vi "Coral Target Loop.vi"(0 "Camera Name":string="cam0") -> ()   [LabVIEW 2023]
uses:
  April Tags/Camera Info.ctl
  State Machine/Coral States.ctl
  State Machine/Coral Main CLuster.ctl
  <vilib>/vision/Image Controls.llb/IMAQ Image.ctl
  Steam Type.ctl
  Ball/State Machine/Ball States.ctl
  Camera Set Up/Event Setup Types.ctl
  <vilib>/Rock Robotics/Network Tables/NT Write String.vi
  <vilib>/Utility/config.llb/Read Key (String).vi
  <vilib>/Utility/config.llb/Write Key (String).vi
  <vilib>/Utility/config.llb/NI_LVConfig.lvlib
  <vilib>/vision/NI_Vision_Development_Module.lvlib
panel:
  in  "Main":enum32{"Page 1", "Page 2"}(tab)
  out "Algae Distance":dbl[](array[numeric]) caption="Distance" format="%.1f"
  out "Algae Angle":dbl[](array[numeric]) caption="Angle" format="%.1f"
  out "Image":T1(plugin-control)
  in  "Settings":bool
  in  "Save":bool
  in  "Tools":bool
  out "Ball Fps":dbl format="%#.0f"
  in  "Home":bool
  in  "FOV":dbl=68.5
  in  "Coral Color Range":T2={"Hue"={21.620689392089844, 69.62068939208984}, "Sat"={66.41378784179688, 255.0}, "Val"={96.0, 255.0}} caption="Color Range" {"Hue" scale=0.0..255.0 scale format="%#_3g"}
  out "Mask":T1(plugin-control)
  in  "Score Threshold %":dbl=80.0
  in  "Robot Calibration Cluster":T3={"Camera Height on robot (in)"=34.5, "Camera Angle on the robot (deg)"=28.3, "Camera FOV Top to Bottom View Angle (deg)"=0.946, "Camera FOV Left to Right View Angle (deg)"=26.5, "Target size (in)"=6.5, "Distance to front of bumper (in)"=9.75, "Focal Length (mm)"=10.0} {"Camera FOV Left to Right View Angle (deg)" format="%#_13g"; "Focal Length (mm)" format="%#_13g"; "Distance to front of bumper (in)" format="%#_13g"; "Target size (in)" format="%#_13g"; "Camera FOV Top to Bottom View Angle (deg)" format="%#_13g"; "Camera Angle on the robot (deg)" format="%#_13g"; "Camera Height on robot (in)" format="%#_13g"}
  # "Edit the camera name to the camera that you are going to use for this target package"
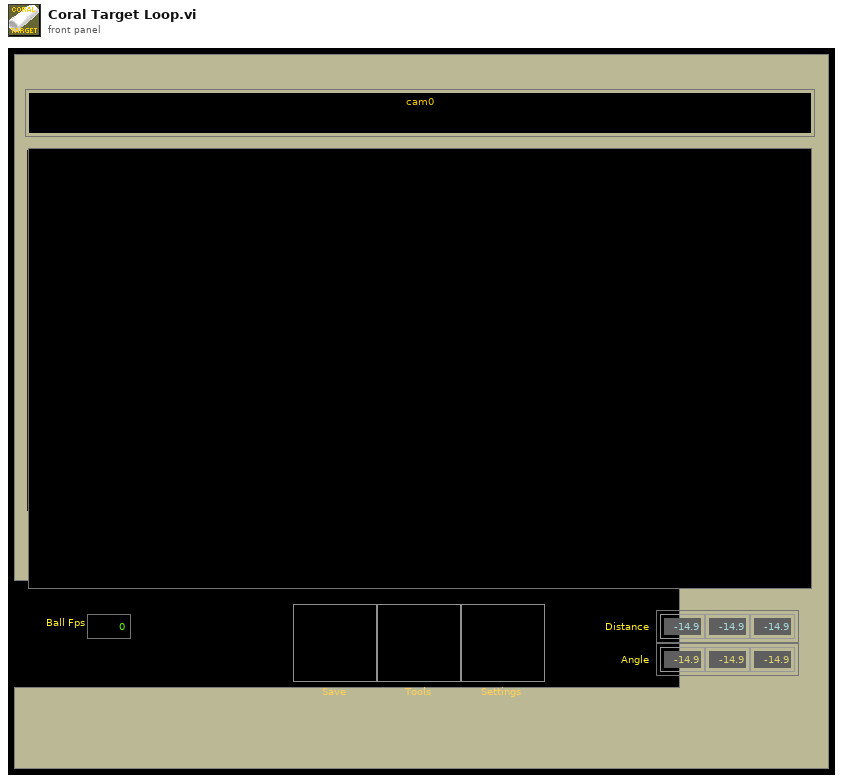
[diagram p1: front panel]
types:
  T1 = typedef "IMAQ Image.ctl" = refnum<image>
  T2 = cluster{"Hue":cluster{dbl, dbl}, "Sat":cluster{dbl, dbl}, "Val":cluster{dbl, dbl}}
  T3 = typedef "Camera Info.ctl" = cluster{"Camera Height on robot (in)":dbl, "Camera Angle on the robot (deg)":dbl, "Camera FOV Top to Bottom View Angle (deg)":dbl, "Camera FOV Left to Right View Angle (deg)":dbl, "Target size (in)":dbl, "Distance to front of bumper (in)":dbl, "Focal Length (mm)":dbl}
  T4 = typedef "Coral Main CLuster.ctl" = cluster{"Coral FIFO":T5[], "Camera Name":string, "Coral path":path, "Control Ref's":refnum<vi>[], "Greyscale Mask Image":T1, "Main Image":T1, "Coral Color Range":cluster{"Hue":cluster{dbl, dbl}, "Sat":cluster{dbl, dbl}, "Val":cluster{dbl, dbl}}, "Timeout":i32}
  T5 = typedef "Coral States.ctl" = enum16{"Message Dispatcher", "INI", "Open", "Save", "Exit"}
  T6 = typedef "Particle Parameters" = i32
  T7 = typedef "Steam Type.ctl" = enum8{"Unknown", "Apriltag", "Algae", "Coral"}
  T8 = typedef "Event Setup Types.ctl" = enum16{"Default", "Camera Loop Started", "Close Settings", "GreyScale", "Open Front Panel", "Save Data", "Exit"}
  T9 = typedef "Ball States.ctl" = enum16{"Message Dispatcher", "INI", "Open", "Save", "Exit"}
  T10 = typedef "Target Fields.ctl" = cluster{"diameter points":cluster{"first point":cluster{"x":dbl, "y":dbl}, "projected point":cluster{"x":dbl, "y":dbl}}, "normalized center":cluster{"x":dbl, "y":dbl}, "Overall Score":dbl, "Area Score":dbl, "Moment Score":dbl, "Aspect Score":dbl, "Distance (ft)":dbl, "Upper Goal":bool}
  T11 = cluster{cluster{"Lower":dbl, "Upper":dbl}, cluster{"Lower":dbl, "Upper":dbl}, cluster{"Lower":dbl, "Upper":dbl}}
  T12 = typedef "Image Type" = u32
  T13 = typedef "NI_LVConfig.lvlib/Config Data RefNum.ctl" = refnum<k1>
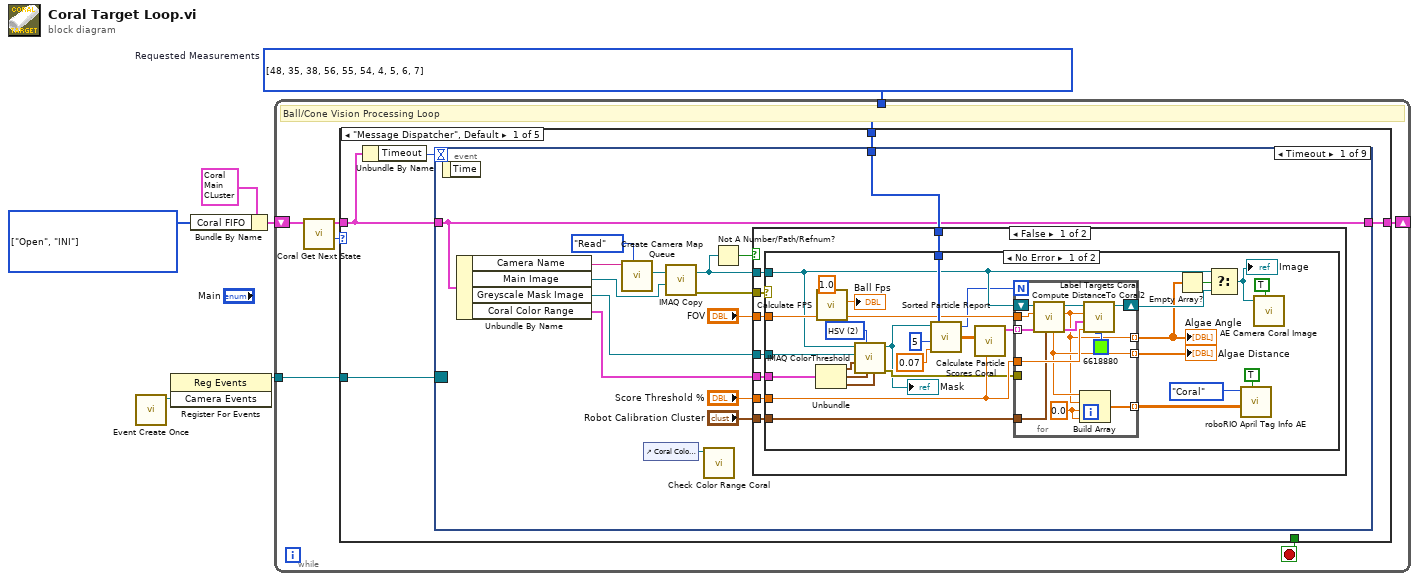
[diagram p0: block diagram]
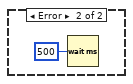
[diagram p2: hidden frame]
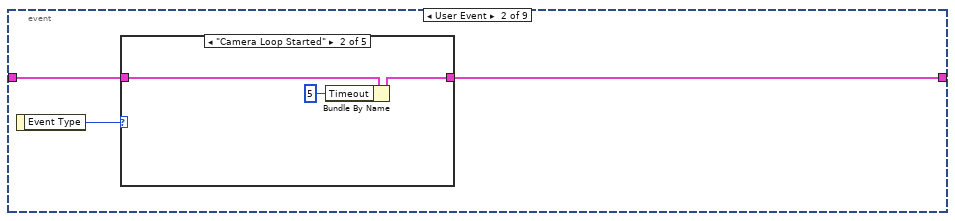
[diagram p4: hidden frame]
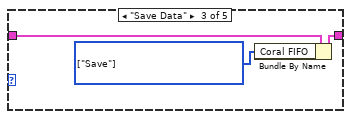
[diagram p6: hidden frame]
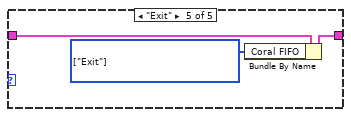
[diagram p8: hidden frame]
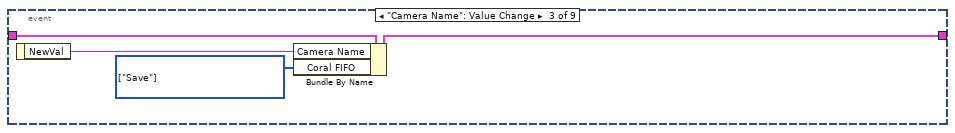
[diagram p9: hidden frame]
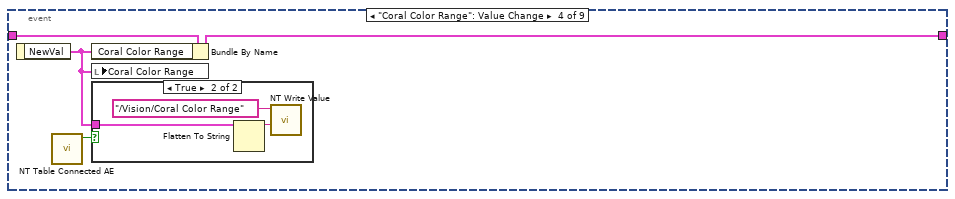
[diagram p10: hidden frame]
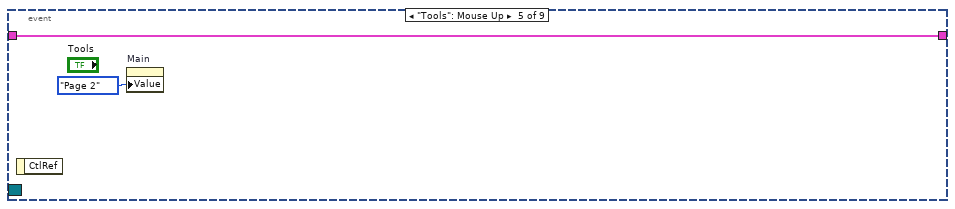
[diagram p12: hidden frame]
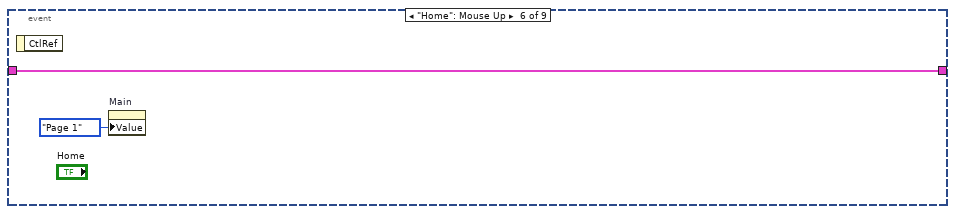
[diagram p13: hidden frame]
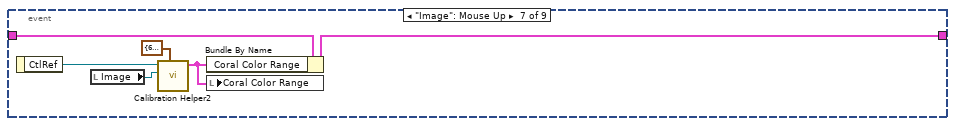
[diagram p14: hidden frame]
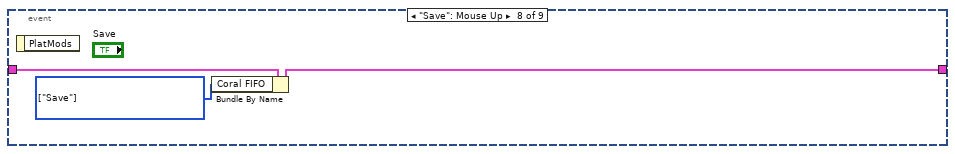
[diagram p15: hidden frame]
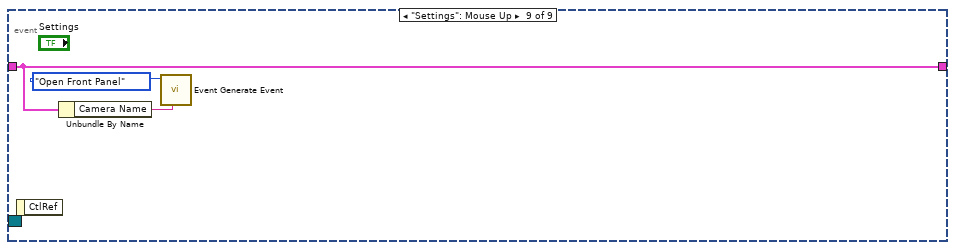
[diagram p16: hidden frame]
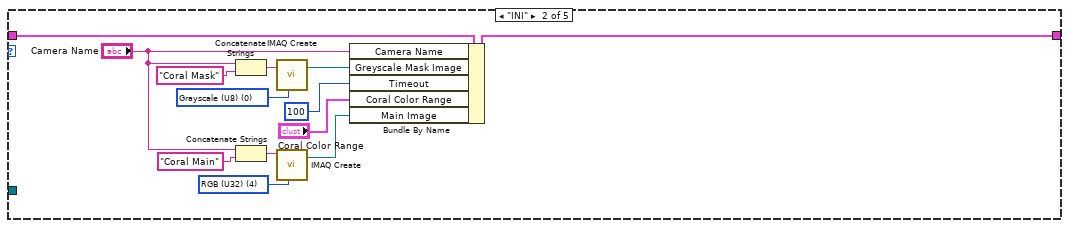
[diagram p17: hidden frame]
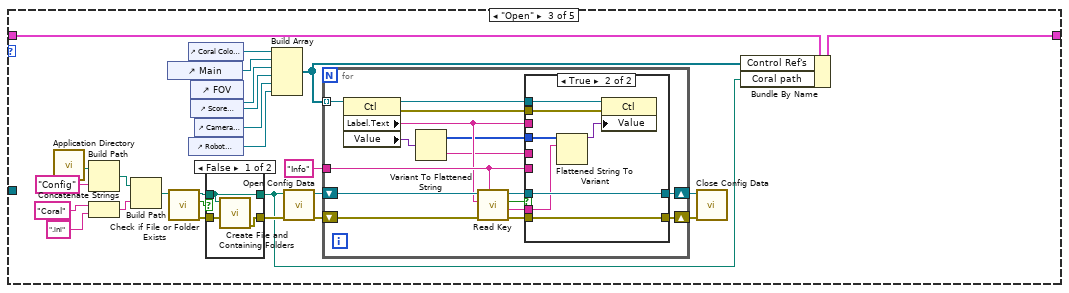
[diagram p18: hidden frame]
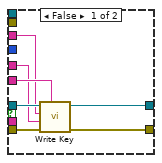
[diagram p20: hidden frame]
diagram:
  w2 = T5[] [enum."Open", enum."INI"] items=["Message Dispatcher", "INI", "Open", "Save", "Exit"] ("Ball FIFO")
  w4 = T6[] [48, 35, 38, 56, 55, 54, 4, 5, 6, 7] items=["Center of Mass X", "Center of Mass Y", "First Pixel X", "First Pixel Y", "Bounding Rect Left", "Bounding Rect Top", "Bounding Rect Right", "Bounding Rect Bottom", "Max Feret Diameter Start X", "Max Feret Diameter Start Y", "Max Feret Diameter End X", "Max Feret Diameter End Y", "Max Horiz. Segment Length Left", "Max Horiz. Segment Length Right", "Max Horiz. Segment Length Row", "-", "Bounding Rect Width", "Bounding Rect Height", "Bounding Rect Diagonal", "Perimeter", "Convex Hull Perimeter", "Holes' Perimeter", "Max Feret Diameter", "Equivalent Ellipse Major Axis", "Equivalent Ellipse Minor Axis", "Equivalent Ellipse Minor Axis (Feret)", "Equivalent Rect Long Side", "Equivalent Rect Short Side", "Equivalent Rect Diagonal", "Equivalent Rect Short Side (Feret)", "Average Horiz. Segment Length", "Average Vert. Segment Length", "Hydraulic Radius", "Waddel Disk Diameter", "-", "Area", "Holes' Area", "Particle & Holes' Area", "Convex Hull Area", "Image Area", "-", "Number of Holes", "Number of Horiz. Segments", "Number of Vert. Segments", "-", "Orientation", "Max Feret Diameter Orientation", "-", "% Area/Image Area", "% Area/(Particle & Holes' Area)", "Ratio of Equivalent Ellipse Axes", "Ratio of Equivalent Rect Sides", "-", "Elongation Factor", "Compactness Factor", "Heywood Circularity Factor", "Type Factor", "-", "Sum X", "Sum Y", "Sum XX", "Sum XY", "Sum YY", "Sum XXX", "Sum XXY", "Sum XYY", "Sum YYY", "-", "Moment of Inertia XX", "Moment of Inertia XY", "Moment of Inertia YY", "Moment of Inertia XXX", "Moment of Inertia XXY", "Moment of Inertia XYY", "Moment of Inertia YYY", "Norm. Moment of Inertia XX", "Norm. Moment of Inertia XY", "Norm. Moment of Inertia YY", "Norm. Moment of Inertia XXX", "Norm. Moment of Inertia XXY", "Norm. Moment of Inertia XYY", "Norm. Moment of Inertia YYY", "Hu Moment 1", "Hu Moment 2", "Hu Moment 3", "Hu Moment 4", "Hu Moment 5", "Hu Moment 6", "Hu Moment 7"]  # Requested Measurements
  n1 = call "Event Create Once.vi"() -> ("Camera Events"=w6:refnum<user-event>)  [unwired: 10 in, 1 out]
  n2 = register-events(w6) -> (reference out=w5:refnum<event-registration>)  [unwired: 2 in, 1 out]
  n3 = Bundle By Name(cluster=T4 {"Coral FIFO"=[], "Camera Name"="", "Coral path"=path "", "Control Ref's"=[], "Greyscale Mask Image"=refnum, "Main Image"=refnum, "Coral Color Range"={"Hue"={21.620689392089844, 69.62068939208984}, "Sat"={66.41378784179688, 255.0}, "Val"={96.0, 255.0}}, "Timeout"=5} ("output cluster"), "Coral FIFO"=w2) -> (w3:T4)
  n4 = while {
    tunnel: w4 -> [w13]
    tunnel: w5 -> [w12]
    shift-right: [w7] -> _
    shift-left: w3 -> [w10]
    stop <- w11 stop-if-true
    # "Ball/Cone Vision Processing Loop"
    n5 = call "Coral Get Next State.vi"("Coral Main Cluster in"=w10) -> ("Next State"=w9:T9, "Coral Main Cluster out"=w8:T4)  [unwired: 9 in]
    n6 = case shown="\"Message Dispatcher\", Default" w9 {
      tunnel: w13 -> [w18 _ _ _ _]
      tunnel: w12 -> [w17 _ _ _ _]
      tunnel: [_ _ _ _ TRUE] -> w11
      tunnel: w8 -> [w15 w135 w149 w202 w219]
      tunnel: [w16 w134 w147 w202 w219] -> w7
      frame "Message Dispatcher", Default {
        n7 = Unbundle By Name(w15) -> ("Timeout"=w14:i32)
        n8 = event shown="[0] Timeout" {
          selector: w17 -> [_ _ _ _ _ _ _ _ _]
          dyn-events: _ -> [_ _ _ _ _ _ _ _ _]
          timeout: w14 -> [_ _ _ _ _ _ _ _ _]
          tunnel: w18 -> [w33 _ _ _ _ _ _ _ _]
          tunnel: w15 -> [w28 w87 w102 w106 w110 w112 w116 w122 w124]
          tunnel: [w28 w85 w101 w105 w110 w112 w115 w121 w124] -> w16
          event Timeout {
            n9 = event-data() -> ()  [unwired: 1 in, 1 out]
            n10 = Unbundle By Name(w28) -> ("Camera Name"=w30:string, "Main Image"=w24:T1, "Greyscale Mask Image"=w29:T1, "Coral Color Range"=w27:T2)
            n11 = call "Create Camera Map Queue.vi"("Action"=enum16{"Read", "Write"}."Read", "Camera"=w30) -> ("Image out"=w25:T1)  [unwired: 8 in, 1 out]
            n12 = control-ref of="Coral Color Range"() -> (w21:refnum<vi>)
            n13 = call "IMAQ Copy"("Image Dst"=w24, "Image Src"=w25) -> ("error out"=w23:errorcluster, "Image Dst Out"=w19:T1)  [unwired: 4 in]
            n14 = call "Check Color Range Coral.vi"("Coral Color Range"=w21) -> ()  [unwired: 11 in]
            n15 = Not A Number/Path/Refnum?(number/path/refnum=w19) -> (NaN/Path/Refnum?=w20:bool)
            n16 = case shown="False" w20 {
              tunnel: w33 -> [w41 _]
              tunnel: "Score Threshold %" -> [w40 _]
              tunnel: w29 -> [w39 _]
              tunnel: w27 -> [w38 _]
              tunnel: "FOV" -> [w37 _]
              tunnel: w19 -> [w36 _]
              tunnel: w23 -> [w35 _]
              tunnel: "Robot Calibration Cluster" -> [w34 _]
              frame False {
                n17 = case shown="No Error" w35 {
                  tunnel: w41 -> [w70 _]
                  tunnel: w39 -> [w68 _]
                  tunnel: w37 -> [w67 _]
                  tunnel: w38 -> [w66 _]
                  tunnel: w40 -> [w65 _]
                  tunnel: w36 -> [w64 _]
                  tunnel: w34 -> [w43 _]
                  frame No Error {
                    w59 = u16 2 items=["RGB", "HSL", "HSV", "HSI"] ("Color Mode")
                    n18 = Unbundle(w66) -> ("Hue"=w54:cluster{dbl, dbl}, "Sat"=w53:cluster{dbl, dbl}, "Val"=w52:cluster{dbl, dbl})
                    n19 = call "Calculate FPS.vi"("Frames Processed"=1.0) -> ("Fps"=→"Ball Fps":dbl)  [unwired: 10 in]
                    n20 = call "IMAQ ColorThreshold"("Blue or Luma or Val or Inten Range"=w52, "Green or Sat Range"=w53, "Color Mode"=w59, "Red or Hue Range"=w54, "Image Dst"=w68, "Image Src"=w64) -> ("error out"=w58:errorcluster, "Image Dst Out"=w42:T1)  [unwired: 4 in]
                    "Mask" <- w42
                    n21 = call "Sorted Particle Report.vi"("Min Area Size %"=0.07 ("Size Limit %"), "Particle Count Limit"=5 ("Particle Count LImit"), "Pixel Measurements"=w70, "Image in"=w42) -> ("Sorted Data"=w62:dbl[][], "Particles"=w57:i32)  [unwired: 1 out]
                    n22 = call "Calculate Particle Scores Coral.vi"("Limit"=w65, "Sorted Data"=w62) -> ("Scores"=w61:T10[])  [unwired: 9 in]
                    n23 = for {
                      N: w57 -> [_]
                      tunnel: w61 -> [w81] mode=indexing
                      shift-right: [w83] -> w56
                      shift-left: w64 -> [w79]
                      tunnel: w65 -> [w82]
                      tunnel: [w74] -> w51 mode=indexing
                      tunnel: w58 -> [_]
                      tunnel: w67 -> [w77]
                      tunnel: [w75] -> w50 mode=indexing
                      tunnel: [w72] -> w44 mode=indexing
                      tunnel: w43 -> [w71]
                      w73 = 0.0 ("element")
                      n24 = call "Compute DistanceTo Coral2.vi"("Robot Calibration Cluster"=w71, "results 2"=w81, "FOV Left to Right (deg)"=w77, "Image Src"=w79) -> ("results out"=w78:T10, "Offset Angle"=w74:dbl, "Image Dst Out"=w80:T1, "Distance from target (in)"=w75:dbl)  [unwired: 4 in]
                      n25 = Build Array(w75, w74, w73, w73) -> (w72:dbl[])
                      n26 = call "Label Targets Coral.vi"("Color"=u32 6618880, "Score Threshold"=w82, "results"=w78, "Angle"=w74, "Image in"=w80) -> ("Image out"=w83:T1)  [unwired: 6 in]
                    }
                    "Algae Angle" <- w51
                    "Algae Distance" <- w50
                    n27 = Empty Array?(array=w51) -> (empty?=w55:bool)
                    n28 = Select(t=w64, s=w55, f=w56) -> (s? t:f=w69:T1)
                    "Image" <- w69
                    n29 = call "roboRIO April Tag Info AE.vi"("Update"=TRUE, "Info in"=w44, "Stream Type"=Steam_Type."Coral") -> ()  [unwired: 8 in, 1 out]
                    n30 = call "AE Camera Coral Image.vi"("Update"=TRUE, "Ball Image in"=w69) -> ()  [unwired: 9 in, 1 out]
                  }
                  frame Error {
                    n31 = Wait (ms)(milliseconds to wait=u32 500) -> ()  [unwired: 1 out]
                  }
                }
              }
              frame True {
              }
            }
          }
          event User Event {
            n32 = event-data() -> ("Event Type"=w86:T8)  [unwired: 1 in]
            n33 = case shown="\"Camera Loop Started\"" w86 {
              tunnel: w87 -> [w88 w91 w94 w95 w98]
              tunnel: [w88 w90 w93 w95 w97] -> w85
              frame "Default", Default {
              }
              frame "Camera Loop Started" {
                n34 = Bundle By Name(cluster=w91, "Timeout"=5) -> (w90:T4)
              }
              frame "Save Data" {
                w92 = T9[] [enum."Save"] items=["Message Dispatcher", "INI", "Open", "Save", "Exit"] ("Ball FIFO")
                n35 = Bundle By Name(cluster=w94, "Coral FIFO"=w92) -> (w93:T4)
              }
              frame "Open Front Panel" {
              }
              frame "Exit" {
                w96 = T9[] [enum."Exit"] items=["Message Dispatcher", "INI", "Open", "Save", "Exit"] ("Ball FIFO")
                n36 = Bundle By Name(cluster=w98, "Coral FIFO"=w96) -> (w97:T4)
              }
            }
          }
          event "Camera Name": Value Change {
            w99 = T9[] [enum."Save"] items=["Message Dispatcher", "INI", "Open", "Save", "Exit"] ("Ball FIFO")
            n37 = event-data() -> ("NewVal"=w100:string)  [unwired: 1 in]
            n38 = Bundle By Name(cluster=w102, "Camera Name"=w100, "Coral FIFO"=w99) -> (w101:T4)
          }
          event "Coral Color Range": Value Change {
            n39 = event-data() -> ("NewVal"=w103:T2)  [unwired: 1 in]
            n40 = call "NT Table Connected AE.vi"() -> ("NT Table Connected out"=w104:bool)  [unwired: 11 in]
            n41 = Bundle By Name(cluster=w106, "Coral Color Range"=w103) -> (w105:T4)
            n42 = local write "Coral Color Range"(w103) -> ()
            n43 = case shown="True" w104 {
              tunnel: w103 -> [_ w107]
              frame False {
              }
              frame True {
                n44 = Flatten To String(anything=w107) -> (data string=w109:string)  [unwired: 3 in, 2 out]
                n45 = call-poly <vilib>:"NT Write Value.vi"("value"=w109, "name"="/Vision/Coral Color Range" ("Name")) -> ()  [unwired: 9 in, 1 out]
              }
            }
          }
          event "Tools": Mouse Up {
            n46 = event-data() -> ()  [unwired: 1 in, 1 out]
            n47 = property on="Main" class="TabCtl (strict)"("Value"=enum32{"Page 1", "Page 2"}."Page 2" ("Main")) -> ()  [unwired: 2 in, 2 out]
          }
          event "Home": Mouse Up {
            n48 = event-data() -> ()  [unwired: 1 in, 1 out]
            n49 = property on="Main" class="TabCtl (strict)"("Value"=enum32{"Page 1", "Page 2"}."Page 1" ("Main")) -> ()  [unwired: 2 in, 2 out]
          }
          event "Image": Mouse Up {
            n50 = event-data() -> ("CtlRef"=w118:refnum<vi>)  [unwired: 1 in]
            n51 = local read "Image"() -> (w117:T1)
            n52 = call "Calibration Helper2.vi"("Std Devs"=cluster{"H":dbl, "S":dbl, "V":dbl} {"H"=6.0, "S"=6.0, "V"=6.0} ("Std Devs Ball"), "Image"=w117, "Image Ctl Refnum"=w118) -> ("output color"=w114:T11)  [unwired: 7 in, 1 out]
            n53 = Bundle By Name(cluster=w116, "Coral Color Range"=w114) -> (w115:T4)
            n54 = local write "Coral Color Range"(w114) -> ()
          }
          event "Save": Mouse Up {
            w120 = T9[] [enum."Save"] items=["Message Dispatcher", "INI", "Open", "Save", "Exit"] ("Ball FIFO")
            n55 = event-data() -> ()  [unwired: 1 in, 1 out]
            n56 = Bundle By Name(cluster=w122, "Coral FIFO"=w120) -> (w121:T4)
          }
          event "Settings": Mouse Up {
            n57 = event-data() -> ()  [unwired: 1 in, 1 out]
            n58 = Unbundle By Name(w124) -> ("Camera Name"=w123:string)
            n59 = call "Event Generate Event.vi"("Camera Name"=w123, "Event Type"=Event_Setup_Types."Open Front Panel") -> ()  [unwired: 10 in]
          }
        }
      }
      frame "INI" {
        w131 = T12 4 items=["Grayscale (U8)", "Grayscale (I16)", "Grayscale (SGL)", "Complex (CSG)", "RGB (U32)", "HSL (U32)", "RGB (U64)", "Grayscale (U16)"] ("Image Type")
        w136 = T12 0 items=["Grayscale (U8)", "Grayscale (I16)", "Grayscale (SGL)", "Complex (CSG)", "RGB (U32)", "HSL (U32)", "RGB (U64)", "Grayscale (U16)"] ("Image Type")
        n60 = Concatenate Strings("Camera Name", "Coral Mask" ("string")) -> (w138:string)
        n61 = Concatenate Strings("Camera Name", "Coral Main" ("string")) -> (w130:string)
        n62 = call "IMAQ Create"("Image Name"=w138, "Image Type"=w136) -> ("New Image"=w133:T1)  [unwired: 2 in, 2 out]
        n63 = call "IMAQ Create"("Image Name"=w130, "Image Type"=w131) -> ("New Image"=w127:T1)  [unwired: 2 in, 2 out]
        n64 = Bundle By Name(cluster=w135, "Camera Name"="Camera Name", "Greyscale Mask Image"=w133, "Timeout"=100, "Coral Color Range"="Coral Color Range", "Main Image"=w127) -> (w134:T4)
      }
      frame "Open" {
        n65 = call <vilib>:"Application Directory.vi"() -> ("Application Directory"=w152:path)
        n66 = Build Path(base path=w152, name or relative path="Config") -> (appended path=w150:path)
        n67 = Concatenate Strings("Coral" ("string"), ".ini" ("name or relative path")) -> (w164:string)
        n68 = Build Path(base path=w150, name or relative path=w164) -> (appended path=w145:path)
        n69 = control-ref of="Main"() -> (w157:refnum<vi>)
        n70 = call <vilib>:"Check if File or Folder Exists.vi"("path"=w145) -> ("error out"=w141:errorcluster, "file or folder exists?"=w143:bool, "dup path"=w144:path)  [unwired: 8 in]
        n71 = control-ref of="Coral Color Range"() -> (w158:refnum<vi>)
        n72 = control-ref of="Robot Calibration Cluster"() -> (w139:refnum<vi>)
        n73 = control-ref of="FOV"() -> (w156:refnum<vi>)
        n74 = control-ref of="Score Threshold %"() -> (w155:refnum<vi>)
        n75 = control-ref of="Camera Name"() -> (w140:refnum<vi>)
        n76 = case shown="False" w143 {
          tunnel: [w167 w168] -> w153
          tunnel: w144 -> [w166 w169]
          tunnel: [w166 w169] -> w142
          tunnel: w141 -> [w165 w168]
          frame False {
            n77 = call <vilib>:"Create File and Containing Folders.vi"("error in (no error)"=w165, "file path"=w166) -> ("error out"=w167:errorcluster)  [unwired: 8 in, 1 out]
          }
          frame True {
          }
        }
        n78 = Build Array(w158, w157, w156, w155, w140, w139) -> (w146:refnum<vi>[])
        n79 = call <vilib>:"Open Config Data.vi"("error in (no error)"=w153, "configuration file path"=w142) -> ("error out"=w159:errorcluster, "refnum"=w163:T13)  [unwired: 7 in, 1 out]
        n80 = for {
          tunnel: "Info" ("Camera Name") -> [w182]
          tunnel: w146 -> [w172] mode=indexing
          shift-right: [w184] -> w162
          shift-left: w163 -> [w185]
          shift-right: [w183] -> w161
          shift-left: w159 -> [w181]
          n81 = property class="Ctl"(reference=w172) -> (reference out=w178:refnum<vi>, error out=w177:errorcluster, "Label.Text"=w175:string, "Value"=w171:variant)  [unwired: 1 in]
          n82 = Variant To Flattened String(Variant=w171) -> (data string=w173:string, 1:w170:i16[])
          n83 = call-poly <vilib>:"Read Key.vi"("section"=w182, "error in (no error)"=w181, "key"=w175, "refnum"=w185) -> ("error out"=w174:errorcluster, "value"=w179:string, "found?"=w180:bool, "refnum out"=w176:T13)  [unwired: 4 in]
          n84 = case shown="True" w180 {
            tunnel: w179 -> [_ w194]
            tunnel: w178 -> [_ w199]
            tunnel: w177 -> [_ w198]
            tunnel: w176 -> [w192 w197]
            tunnel: w182 -> [w191 _]
            tunnel: w175 -> [w190 _]
            tunnel: [w189 w197] -> w184
            tunnel: w174 -> [w188 w196]
            tunnel: [w187 w196] -> w183
            tunnel: w173 -> [w186 _]
            tunnel: w170 -> [_ w193]
            frame False {
              n85 = call-poly <vilib>:"Write Key.vi"("section"=w191, "error in (no error)"=w188, "value"=w186, "key"=w190, "refnum"=w192) -> ("error out"=w187:errorcluster, "refnum out"=w189:T13)  [unwired: 4 in, 1 out]
            }
            frame True {
              n86 = Flattened String To Variant(6:w194, 7:w193) -> (3:w195:variant)  [unwired: 1 in, 1 out]
              n87 = property class="Ctl"(reference=w199, error in=w198, "Value"=w195) -> ()  [unwired: 2 out]
            }
          }
        }
        n88 = call <vilib>:"Close Config Data.vi"("error in (no error)"=w161, "refnum"=w162) -> ()  [unwired: 8 in, 2 out]
        n89 = Bundle By Name(cluster=w149, "Control Ref's"=w146, "Coral path"=w142) -> (w147:T4)
      }
      frame "Save" {
        n90 = Unbundle By Name(w202) -> ("Control Ref's"=w200:refnum<vi>[], "Coral path"=w201:path)
        n91 = call <vilib>:"Open Config Data.vi"("configuration file path"=w201) -> ("error out"=w206:errorcluster, "refnum"=w207:T13)  [unwired: 8 in, 1 out]
        n92 = for {
          tunnel: w200 -> [w217] mode=indexing
          tunnel: w207 -> [w216]
          tunnel: w206 -> [w215]
          tunnel: "Info" ("Camera Name") -> [w211]
          tunnel: [w209] -> w205
          tunnel: [w208] -> w204
          n93 = property class="Ctl"(reference=w217, error in=w215) -> (error out=w212:errorcluster, "Label.Text"=w214:string, "Value"=w213:variant)  [unwired: 1 out]
          n94 = Variant To Flattened String(Variant=w213) -> (data string=w210:string)  [unwired: 1 out]
          n95 = call-poly <vilib>:"Write Key.vi"("section"=w211, "error in (no error)"=w212, "value"=w210, "key"=w214, "refnum"=w216) -> ("error out"=w209:errorcluster, "refnum out"=w208:T13)  [unwired: 4 in, 1 out]
        }
        n96 = call <vilib>:"Close Config Data.vi"("error in (no error)"=w205, "refnum"=w204) -> ()  [unwired: 8 in, 2 out]
      }
      frame "Exit" {
        n97 = Unbundle By Name(w219) -> ("Greyscale Mask Image"=w221:T1, "Main Image"=w220:T1)
        n98 = call "IMAQ Dispose"("Image"=w221) -> ()  [unwired: 5 in, 1 out]
        n99 = call "IMAQ Dispose"("Image"=w220) -> ()  [unwired: 5 in, 1 out]
      }
    }
  }
